vi "MALTCON two-hand ctrl status.vi"() -> ()   [LabVIEW 2018]
uses:
  <instrlib>/AltonTech MALT/AltonTech MALT200817.lvlib
panel:
  out "Local Port":u16
  in  "Address":i32=1
  out "Two-Hand Ctrtl Status":bool
  in  "stop":bool
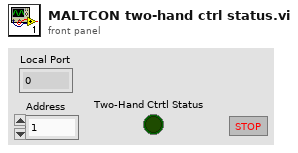
[diagram p1: front panel]
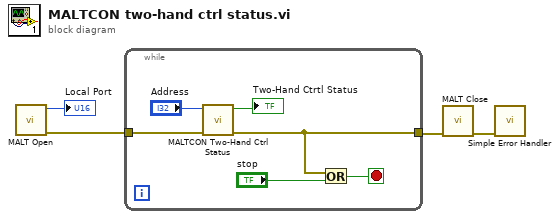
[diagram p0: block diagram]
diagram:
  n1 = call <instrlib>:"MALT Open.vi"() -> ("error out"=w4:errorcluster, "Local Port"=→"Local Port":u16)  [unwired: 10 in]
  n2 = while {
    tunnel: w4 -> [w10]
    tunnel: [w5] -> w3
    stop <- w6 stop-if-true
    n3 = call <instrlib>:"MALTCON Two-Hand Ctrl Status.vi"("error in"=w10, "Address"="Address") -> ("error out"=w5:errorcluster, "Status"=→"Two-Hand Ctrtl Status":bool)  [unwired: 8 in]
    n4 = Or(x=w5, y="stop") -> (x .or. y?=w6:bool)
  }
  n5 = call <instrlib>:"MALT Close.vi"("error in"=w3) -> ("error out"=w2:errorcluster)  [unwired: 10 in]
  n6 = call <vilib>:"Simple Error Handler.vi"("error in (no error)"=w2) -> ()  [unwired: 4 in, 5 out]
